vi "Depth-First-Search.vi"(8 "Tag In":string, 11 "Tree in":refnum<class "Tree.lvclass">) -> (3 "Tree out":refnum<class "Tree.lvclass">)   [LabVIEW 2024, in "Tree.lvclass"]
doc: "This is the Recursive Function \nThat Read All Child Items of The Tag\n(Not including the Item It's Self)\nAfter the operation, the multi items \nwill fill with ALL child items\n\nAnd BE NOTICED!!\nthe single items will fill with the last \nChild Item, not the Tag Item itself"
uses:
  Tree.lvclass
  Tree.lvclass/Tree.ctl
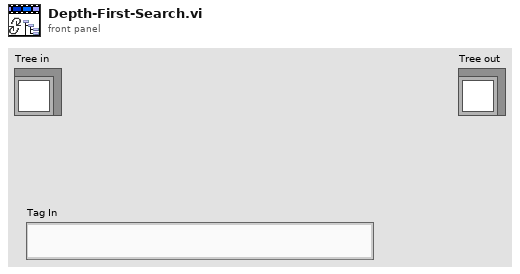
[diagram p1: front panel]
types:
  T1 = typedef "Tree Item.ctl" = cluster{"Parent Tag":string, "Tag":string, "Left Cell":string, "Cells Text":string[], "BFS Index":i32[], "Graph Index":i32, "Item Indent":i32}
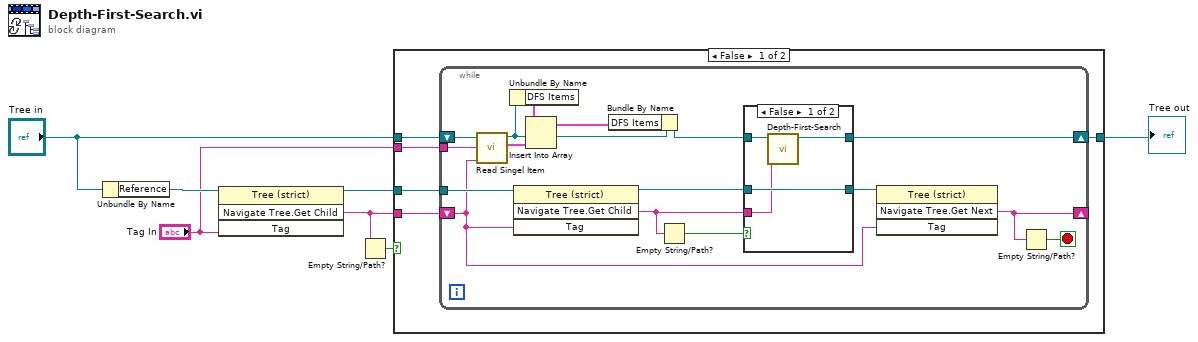
[diagram p0: block diagram]
diagram:
  n1 = Unbundle By Name("Tree in") -> ("Reference"=w7:refnum<vi>)
  n2 = invoke class="Tree (strict)" method="Navigate Tree.Get Child"(reference=w7, "Tag"="Tag In") -> (reference out=w3:refnum<vi>, "Navigate Tree:Get Child"=w2:string)  [unwired: 2 in, 2 out]
  n3 = Empty String/Path?(string/path=w2) -> (empty?=w6:bool)
  n4 = case shown="False" w6 {
    tunnel: "Tree in" -> [w10 w35]
    tunnel: [w9 w35] -> w4
    tunnel: w3 -> [w12 _]
    tunnel: w2 -> [w11 _]
    tunnel: "Tag In" -> [w8 _]
    frame False {
      n5 = while {
        shift-right: [w26] -> w9
        shift-left: w10 -> [w24]
        tunnel: w8 -> [w23]
        shift-right: [w15] -> _
        shift-left: w11 -> [w16]
        tunnel: w12 -> [w28]
        stop <- w14 stop-if-true
        n6 = call "Read Singel Item.vi"("Tag"=w16, "Parent Tag"=w23, "Tree in"=w24) -> ("Element Out"=w21:T1, "Tree out"=w20:refnum<class "Tree.lvclass">)  [unwired: 7 in]
        n7 = Unbundle By Name(w20) -> ("DFS Items"=w22:T1[])
        n8 = invoke class="Tree (strict)" method="Navigate Tree.Get Child"(reference=w28, "Tag"=w16) -> (reference out=w25:refnum<vi>, "Navigate Tree:Get Child"=w13:string)  [unwired: 2 in, 2 out]
        n9 = Insert Into Array(array=w22, new element=w21) -> (w19:T1[])  [unwired: 1 in]
        n10 = Bundle By Name(cluster=w20, "DFS Items"=w19) -> (w18:refnum<class "Tree.lvclass">)
        n11 = Empty String/Path?(string/path=w13) -> (empty?=w27:bool)
        n12 = case shown="False" w27 {
          tunnel: w18 -> [w31 w34]
          tunnel: [w30 w34] -> w26
          tunnel: w25 -> [w32 w33]
          tunnel: [w32 w33] -> w17
          tunnel: w13 -> [w29 _]
          frame False {
            n13 = call "Depth-First-Search.vi"("Tag In"=w29, "Tree in"=w31) -> ("Tree out"=w30:refnum<class "Tree.lvclass">)  [unwired: 9 in]
          }
          frame True {
          }
        }
        n14 = invoke class="Tree (strict)" method="Navigate Tree.Get Next"(reference=w17, "Tag"=w16) -> ("Navigate Tree:Get Next Item"=w15:string)  [unwired: 2 in, 3 out]
        n15 = Empty String/Path?(string/path=w15) -> (empty?=w14:bool)
      }
    }
    frame True {
    }
  }
  "Tree out" <- w4
